vi "GEA2 Serial Check CRC.vi"(8 "error in (no error)":errorcluster, 10 "CRCArray":u8[](array[numeric]), 11 "CRCRead in":u8[](array[numeric])) -> (0 "error out":errorcluster, 3 "CRC Match":bool)   [LabVIEW 2014]
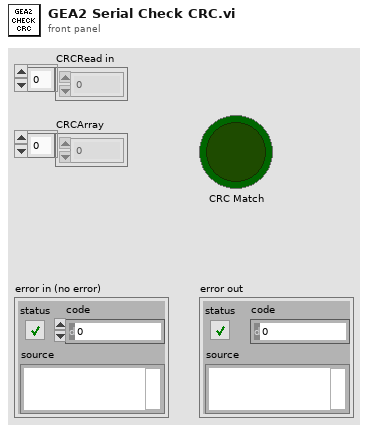
[diagram p1: front panel]
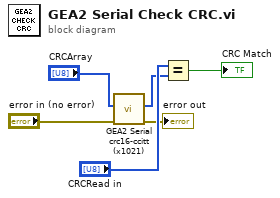
[diagram p0: block diagram]
diagram:
  n1 = call "GEA2 Serial crc16-ccitt (x1021).vi"("error in (no error)"="error in (no error)", "unsigned byte array"="CRCArray") -> ("error out (dup)"=→"error out":errorcluster, "CRC"=w3:u8[])  [unwired: 8 in]
  n2 = Equal?(x="CRCRead in", y=w3) -> (x = y?=→"CRC Match":bool)
